vi "set_triggered.vi"(8 "error in (no error)":errorcluster, 10 "triggered?":bool, 11 "GenericScanHead.lvclass in":refnum<class "GenericScanHead.lvclass">) -> (0 "error out":errorcluster, 3 "GenericScanHead.lvclass out":refnum<class "GenericScanHead.lvclass">)   [LabVIEW 2010, in "GenericScanHead.lvclass"]
uses:
  GenericScanHead.lvclass
  GenericScanHead.lvclass/GenericScanHead.ctl
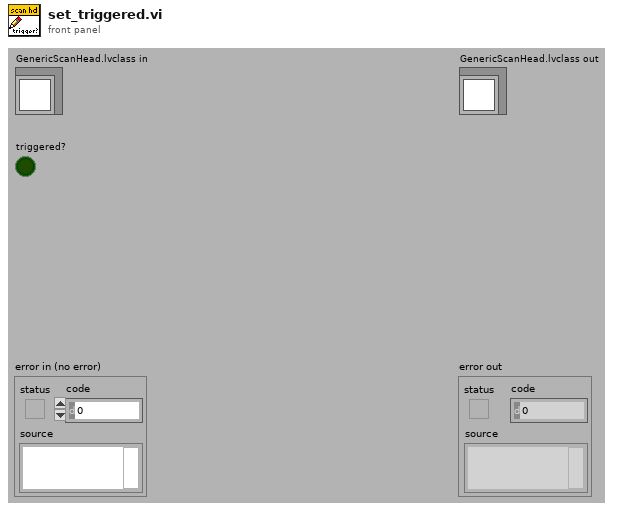
[diagram p1: front panel]
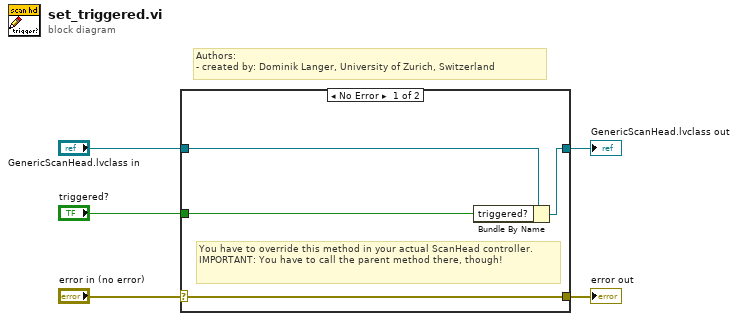
[diagram p0: block diagram]
diagram:
  # "Authors: \n- created by: Dominik Langer, University of Zurich, Switzerland"
  n1 = case shown="No Error" "error in (no error)" {
    selector: "error in (no error)" -> [w9 w10]
    tunnel: [w9 w10] -> w4
    tunnel: [w7 w11] -> w2
    tunnel: "GenericScanHead.lvclass in" -> [w8 w11]
    tunnel: "triggered?" -> [w6 _]
    frame No Error {
      # "You have to override this method in your actual ScanHead controller. \nIMPORTANT: You have to call the parent method there, though!"
      n2 = Bundle By Name(cluster=w8, "triggered?"=w6) -> (w7:refnum<class "GenericScanHead.lvclass">)
    }
    frame Error {
    }
  }
  "error out" <- w4
  "GenericScanHead.lvclass out" <- w2
